vi "test_alignLeftValidationIgnoringLabels.vi"(11 "Test Case In":refnum<class "AlignmentTests.lvclass">) -> (0 "error out":errorcluster, 3 "Test Case Out":refnum<class "AlignmentTests.lvclass">)   [LabVIEW 2023, in "AlignmentTests.lvclass"]
uses:
  AlignmentTests.lvclass
  <vilib>/Astemes/LUnit/Test Case.lvclass/Test Case.ctl
  <vilib>/Astemes/LUnit/Core/LUnit Test Case/Private/Append Fail Result.vi
  <vilib>/Astemes/LUnit/Core/LUnit Test Case/Private/Append Pass Result.vi
  <vilib>/Astemes/LUnit/Core/LUnit Test Case/Private/Run In UI.vi
  <vilib>/Utility/error.llb/Clear Errors.vi
  <vilib>/Astemes/LUnit/Test Case.lvclass
  source/TLC_Geometry.lvlib
panel:
  in  "Numeric 3":dbl
  in  "Numeric 2_long caption":dbl caption="Numeric 2_long catption"
  in  "Numeric 1 long caption":dbl caption="Numeric sdsad"
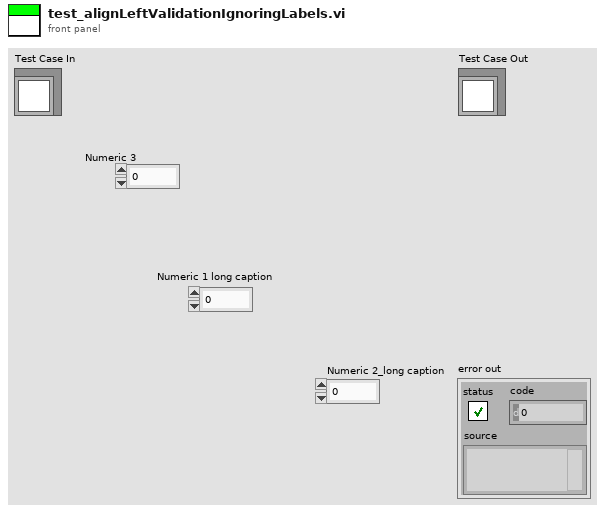
[diagram p1: front panel]
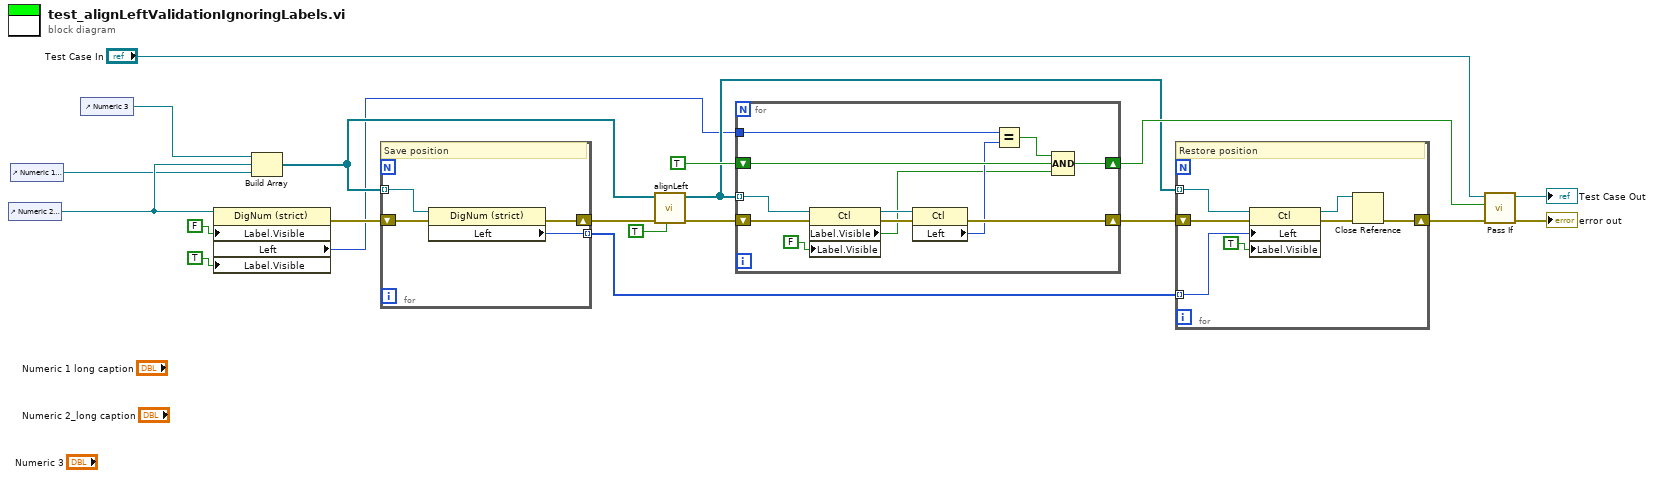
[diagram p0: block diagram]
diagram:
  n1 = control-ref of="Numeric 2_long caption"() -> (w16:refnum<vi>)
  n2 = control-ref of="Numeric 1 long caption"() -> (w15:refnum<vi>)
  n3 = control-ref of="Numeric 3"() -> (w17:refnum<vi>)
  n4 = property class="DigNum (strict)"(reference=w16, "Label.Visible"=FALSE, "Label.Visible"=TRUE) -> (error out=w11:errorcluster, "Left"=w4:i32)  [unwired: 1 in, 1 out]
  n5 = Build Array(w17, w16, w15) -> (w6:refnum<vi>[])
  n6 = for {
    tunnel: w6 -> [w24] mode=indexing
    shift-right: [w22] -> w10
    shift-left: w11 -> [w23]
    tunnel: [w21] -> w7 mode=indexing
    # "Save position"
    n7 = property class="DigNum (strict)"(reference=w24, error in=w23) -> (error out=w22:errorcluster, "Left"=w21:i32)  [unwired: 1 out]
  }
  n8 = call "alignLeft.vi"("useControlBodyOnly"=TRUE ("ignoreCaption&Labels"), "error in (no error)"=w10, "refs"=w6) -> ("error out"=w12:errorcluster, "refs(dup)"=w5:refnum<vi>[])  [unwired: 7 in]
  n9 = for {
    tunnel: w5 -> [w27] mode=indexing
    tunnel: w4 -> [w36]
    shift-right: [w34] -> w13
    shift-left: TRUE -> [w33]
    shift-right: [w32] -> w8
    shift-left: w12 -> [w30]
    n10 = property class="Ctl"(reference=w27, error in=w30, "Label.Visible"=FALSE) -> (reference out=w28:refnum<vi>, error out=w29:errorcluster, "Label.Visible"=w26:bool)
    n11 = property class="Ctl"(reference=w28, error in=w29) -> (error out=w32:errorcluster, "Left"=w31:i32)  [unwired: 1 out]
    n12 = Equal?(x=w36, y=w31) -> (x = y?=w35:bool)
    n13 = Compound Arithmetic op=AND(w35, w33, w26) -> (w34:bool)
  }
  n14 = for {
    tunnel: w5 -> [w43] mode=indexing
    shift-right: [w39] -> w9
    shift-left: w8 -> [w42]
    tunnel: w7 -> [w40] mode=indexing
    # "Restore position"
    n15 = property class="Ctl"(reference=w43, error in=w42, "Left"=w40, "Label.Visible"=TRUE) -> (reference out=w38:refnum<vi>, error out=w41:errorcluster)
    n16 = Close Reference(reference=w38, error in (no error)=w41) -> (error out=w39:errorcluster)
  }
  n17 = call <vilib>:"Pass If.vi"("error in (no error)"=w9, "Pass?"=w13, "LUnit Test Case In"="Test Case In") -> ("error out"=→"error out":errorcluster, "LUnit Test Case Out"=→"Test Case Out":refnum<class "AlignmentTests.lvclass">)  [unwired: 7 in]
